vi "Configure Trigger Level.vi"(6 "Trigger Level 2 (0.0 V)":dbl, 8 "error in (no error)":errorcluster, 9 "Trigger Level 1 (0.0 V)":dbl, 10 "Channel (0: Channel 1)":u16(ring) items=["Channel 1", "Channel 2", "Channel 3", "Channel 4", "Ext", "Ext10"], 11 "VISA resource name":refnum<visa-resource-name>) -> (0 "error out":errorcluster, 3 "VISA resource name out":refnum<visa-resource-name>)   [LabVIEW 2018, in "LeCroy Wave Series.lvlib"]
doc: "This adjusts the trigger level of the specified trigger source."
uses:
  LeCroy Wave Series.lvlib
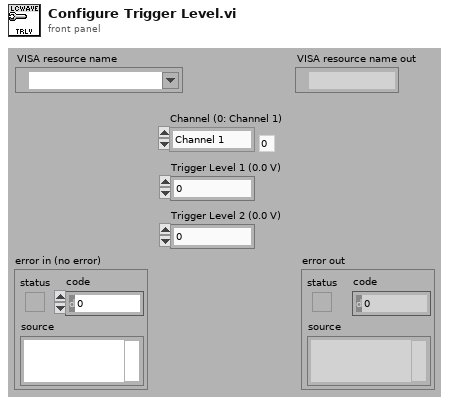
[diagram p1: front panel]
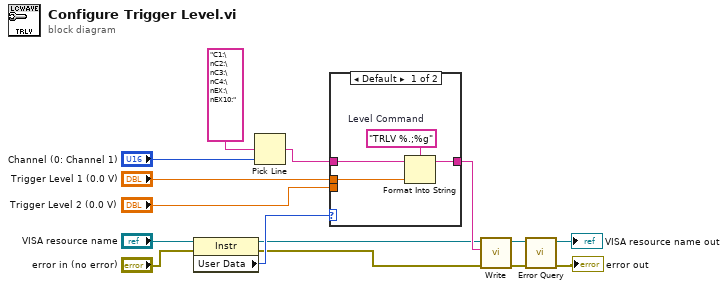
[diagram p0: block diagram]
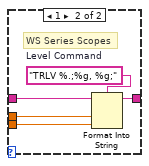
[diagram p2: hidden frame]
diagram:
  n1 = property class="Instr"(reference="VISA resource name", error in="error in (no error)") -> (reference out=w1:refnum<visa-resource-name>, error out=w2:errorcluster, "User Data"=w3:u32)
  n2 = Pick Line(multi-line string="C1:\nC2:\nC3:\nC4:\nEX:\nEX10:", line index="Channel (0: Channel 1)") -> (output string=w14:string)  [unwired: 1 in]
  n3 = case shown="Default" w3 {
    tunnel: w14 -> [w18 w23]
    tunnel: [w17 w22] -> w13
    tunnel: "Trigger Level 1 (0.0 V)" -> [w16 w21]
    tunnel: "Trigger Level 2 (0.0 V)" -> [_ w20]
    frame Default {
      w19 = "TRLV %.;%g"  # Level Command
      n4 = Format Into String(format string=w19, initial string=w18, w16) -> (resulting string=w17:string)  [unwired: 1 in, 1 out]
    }
    frame 1 {
      w24 = "TRLV %.;%g, %g;"  # Level Command
      # "WS Series Scopes"
      n5 = Format Into String(format string=w24, initial string=w23, w21, w20) -> (resulting string=w22:string)  [unwired: 1 in, 1 out]
    }
  }
  n6 = call "Write.vi"("error in (no error)"=w2, "Write Buffer"=w13, "VISA resource name"=w1) -> ("error out"=w10:errorcluster, "VISA resource name out"=w12:refnum<visa-resource-name>)  [unwired: 7 in]
  n7 = call "Error Query.vi"("error in (no error)"=w10, "VISA resource name"=w12) -> ("error out"=→"error out":errorcluster, "VISA resource name out"=→"VISA resource name out":refnum<visa-resource-name>)  [unwired: 6 in, 2 out]
